vi "Initialize.vi"(8 "error in (no error)":errorcluster, 10 "Internal?":bool, 11 "Lauda Settings":T1) -> (0 "error out":errorcluster, 2 "Connection Error":bool, 3 "Lauda Settings":T1)   [LabVIEW 2018, in "Lauda TCU.lvlib"]
uses:
  Lauda TCU.lvlib
  Lauda Settings.ctl
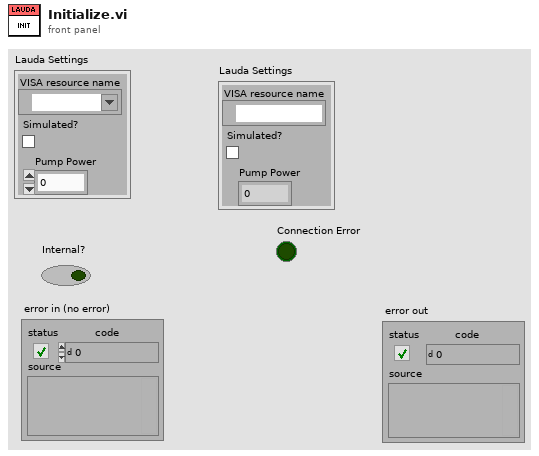
[diagram p1: front panel]
types:
  T1 = typedef "Lauda TCU.lvlib/Lauda Settings.ctl" = cluster{"VISA resource name":refnum<visa-resource-name>, "Simulated?":bool, "Pump Power":i32}
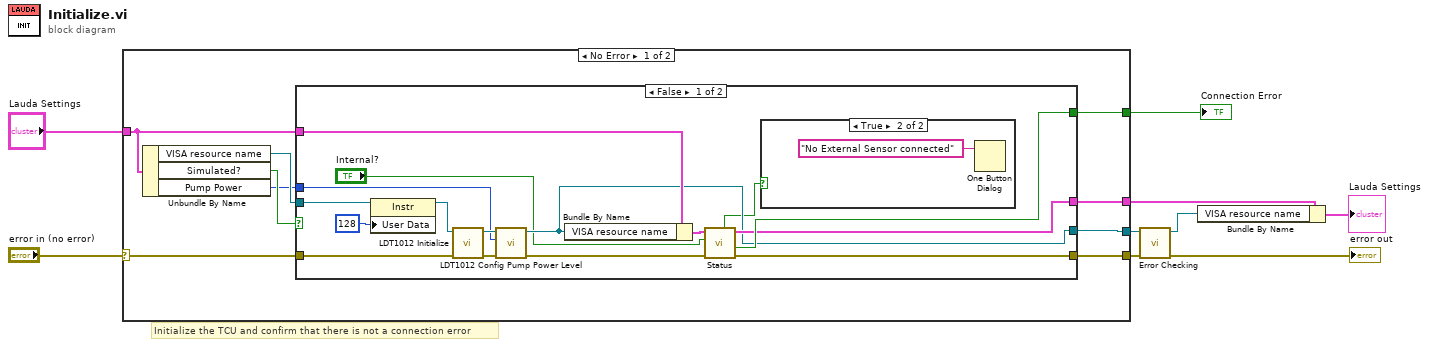
[diagram p0: block diagram]
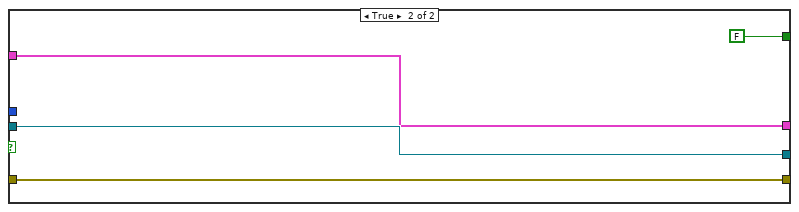
[diagram p3: hidden frame]
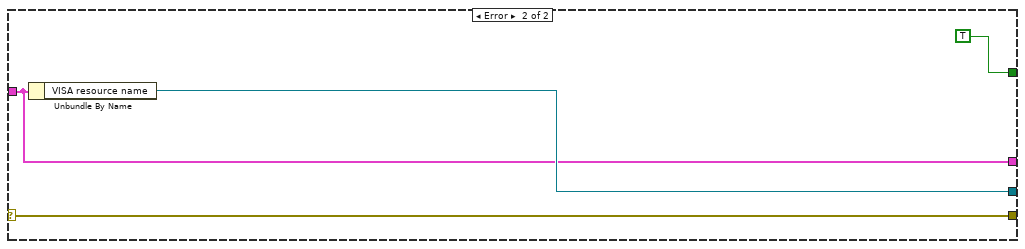
[diagram p4: hidden frame]
diagram:
  # "Initialize the TCU and confirm that there is not a connection error"
  n1 = case shown="No Error" "error in (no error)" {
    selector: "error in (no error)" -> [w18 w43]
    tunnel: "Lauda Settings" -> [w12 w40]
    tunnel: [w17 w43] -> w7
    tunnel: [w15 w42] -> w8
    tunnel: [w13 TRUE] -> w3
    tunnel: [w11 w40] -> w2
    frame No Error {
      n2 = Unbundle By Name(w12) -> ("VISA resource name"=w16:refnum<visa-resource-name>, "Simulated?"=w14:bool, "Pump Power"=w10:i32)
      n3 = case shown="False" w14 {
        tunnel: w18 -> [w31 w39]
        tunnel: [w32 w39] -> w17
        tunnel: [w25 w38] -> w15
        tunnel: w16 -> [w22 w38]
        tunnel: [w34 FALSE] -> w13
        tunnel: w12 -> [w30 w36]
        tunnel: [w33 w36] -> w11
        tunnel: w10 -> [w27 _]
        frame False {
          n4 = property class="Instr"(reference=w22, "User Data"=u32 128 ("General Settings:User Data")) -> (reference out=w20:refnum<visa-resource-name>)  [unwired: 1 in, 1 out]
          n5 = call "LDT1012 Initialize.vi"("error in (no error)"=w31, "VISA resource name"=w20) -> ("error out"=w26:errorcluster, "VISA session"=w28:refnum<visa-resource-name>)  [unwired: 6 in, 2 out]
          n6 = call "LDT1012 Config Pump Power Level.vi"("error in (no error)"=w26, "Pump Power Level (2: Default)"=w27, "VISA session"=w28) -> ("error out"=w24:errorcluster, "dup VISA session"=w25:refnum<visa-resource-name>)  [unwired: 7 in]
          n7 = Bundle By Name(cluster=w30, "VISA resource name"=w25) -> (w29:T1)
          n8 = call "Status.vi"("error in (no error)"=w24, "Internal?"="Internal?", "Lauda Settings"=w29) -> ("error out"=w32:errorcluster, "Connection Error"=w34:bool, "Lauda Settings"=w33:T1, "No external Sensor"=w19:bool)  [unwired: 2 in, 3 out]
          n9 = case shown="True" w19 {
            frame False {
            }
            frame True {
              n10 = One Button Dialog(message="No External Sensor connected") -> ()  [unwired: 1 in, 1 out]
            }
          }
        }
        frame True {
        }
      }
    }
    frame Error {
      n11 = Unbundle By Name(w40) -> ("VISA resource name"=w42:refnum<visa-resource-name>)
    }
  }
  "Connection Error" <- w3
  n12 = call "Error Checking.vi"("error in (no error)"=w7, "VISA resource name"=w8) -> ("error out"=→"error out":errorcluster, "VISA resource name"=w5:refnum<visa-resource-name>)  [unwired: 7 in, 1 out]
  n13 = Bundle By Name(cluster=w2, "VISA resource name"=w5) -> (→"Lauda Settings":T1)
